vi "WFT Get Device Count.vi"(8 "Error In":errorcluster, 10 "Enum Filter":i32(ring) items=["enumfilterAll", "enumfilterEExplorer", "enumfilterDiscovery", "enumfilterDiscovery2", "enumfilterDDiscovery"]) -> (0 "Error Out":errorcluster, 1 "pcDevice":i32, 2 "ret":i32)   [LabVIEW 2020, in "lv_waveforms_toolkit.lvlib"]
uses:
  lv_waveforms_toolkit.lvlib
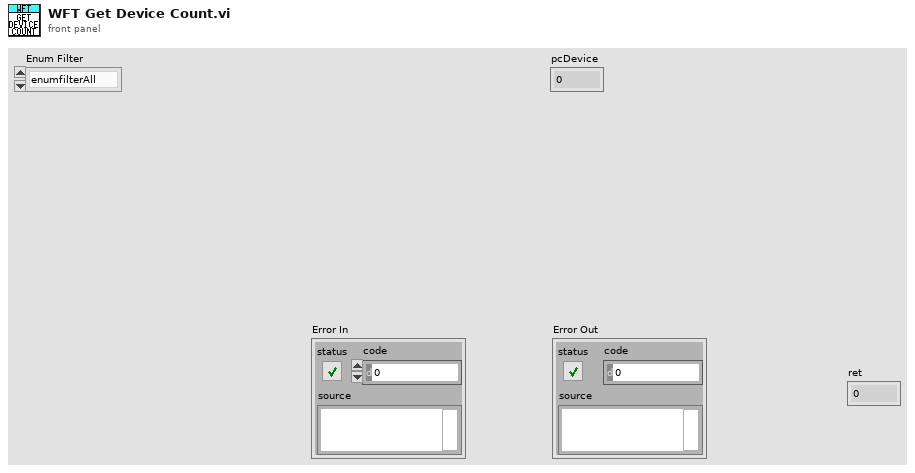
[diagram p1: front panel]
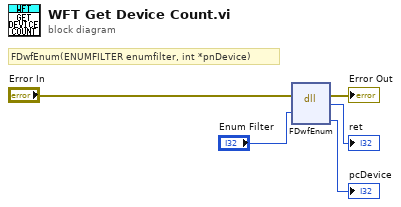
[diagram p0: block diagram]
diagram:
  # "FDwfEnum(ENUMFILTER enumfilter, int *pnDevice)"
  n1 = dll-call lib="dwf" fn="FDwfEnum"(error in="Error In", "enumfilter"="Enum Filter") -> (error out=→"Error Out":errorcluster, "return type"=→"ret":i32, "pcDevice"=→"pcDevice":i32)  [unwired: 4 in, 1 out]
